vi "Get Step Timing in Seconds.vi"(8 "error in (no error)":errorcluster, 11 "Step Index":i32) -> (0 "error out":errorcluster, 3 "Timing":i32)   [LabVIEW 2015, in "UI Handler.lvclass"]
uses:
  UI Handler.lvclass
  UI Handler.lvclass/UI Handler.ctl
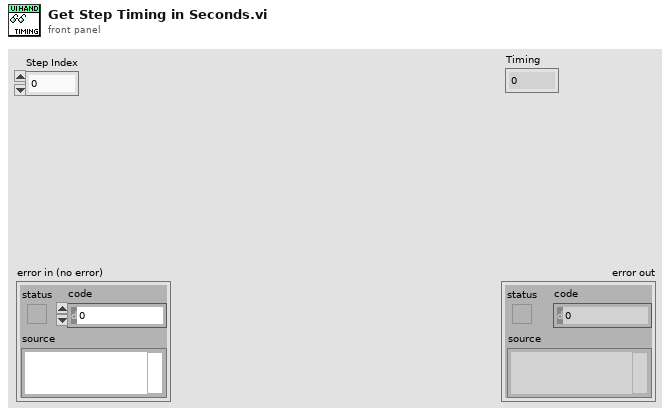
[diagram p1: front panel]
types:
  T1 = typedef "UI Handler.lvclass/Session Handle.ctl" = refnum<data-value>
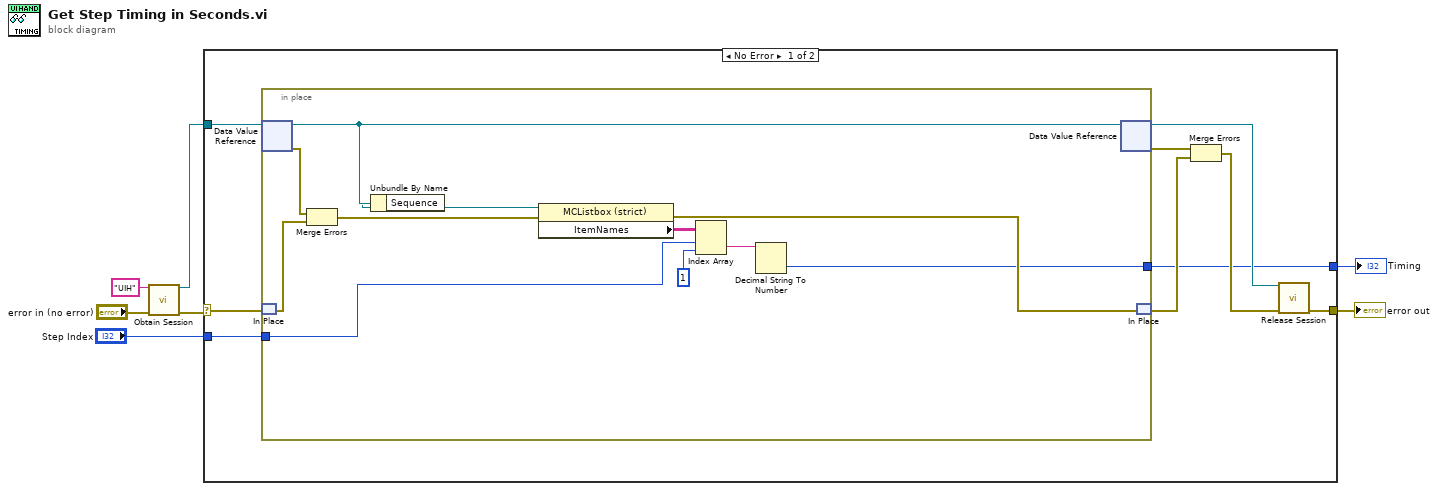
[diagram p0: block diagram]
diagram:
  n1 = call "Obtain Session.vi"("Session  Name ()"="UIH", "error in (no error)"="error in (no error)") -> ("Session Handle"=w3:T1, "error out"=w4:errorcluster)  [unwired: 12 in]
  n2 = case shown="No Error" w4 {
    selector: w4 -> [w13 w28]
    tunnel: w3 -> [w16 _]
    tunnel: [w10 w28] -> w6
    tunnel: "Step Index" -> [w12 _]
    tunnel: [w8 _] -> w1
    frame No Error {
      n3 = in-place {
        in-place-border: w12 -> [w20]
        in-place-border: [w17] -> w8
        n4 = in-place-dvr #1(w16) -> (w27:refnum<class "UI Handler.lvclass">, w22:errorcluster)
        n5 = in-place-match #2(w13) -> (w21:errorcluster)
        n6 = Merge Errors(w22, w21) -> (w23:errorcluster)
        n7 = Unbundle By Name(w27) -> ("Sequence"=w24:refnum<vi>)
        n8 = property on="Property Node" class="MCListbox (strict)"(reference=w24, error in=w23) -> (error out=w19:errorcluster, "ItemNames"=w26:string[][])  [unwired: 1 out]
        n9 = Index Array(array=w26, index (row)=w20, index (col)=1 ("disabled index (col)")) -> (element=w18:string)
        n10 = Decimal String To Number(string=w18) -> (number=w17:i32)  [unwired: 2 in, 1 out]
        n11 = in-place-dvr #1(w27) -> (w9:T1, w14:errorcluster)
        n12 = in-place-match #2(w19) -> (w15:errorcluster)
      }
      n13 = Merge Errors(w14, w15) -> (w11:errorcluster)
      n14 = call "Release Session.vi"("Session Handle"=w9, "error in (no error)"=w11) -> ("error out"=w10:errorcluster)  [unwired: 13 in]
    }
    frame Error {
    }
  }
  "error out" <- w6
  "Timing" <- w1
